vi "Sigma_SetSpeed.vi"(0 "VISA resource name":refnum<visa-resource-name>, 1 "Travel per Pulse (0.004mm)":dbl=0.004, 2 "Min (1mm) 2":dbl=1.0, 3 "Max (2mm) 2":dbl=2.0, 4 "Rate (1mm) 2":dbl=1.0, 5 "error in (no error)":errorcluster, 6 "Axis (1)":string="1", 8 "Min (1mm)":dbl=1.0, 10 "Max (2mm)":dbl=2.0, 12 "Rate (1mm)":dbl=1.0) -> (14 "VISA resource name out":refnum<visa-resource-name>, 19 "error out":errorcluster)   [LabVIEW 2018]
panel:
  out "resulting string":string
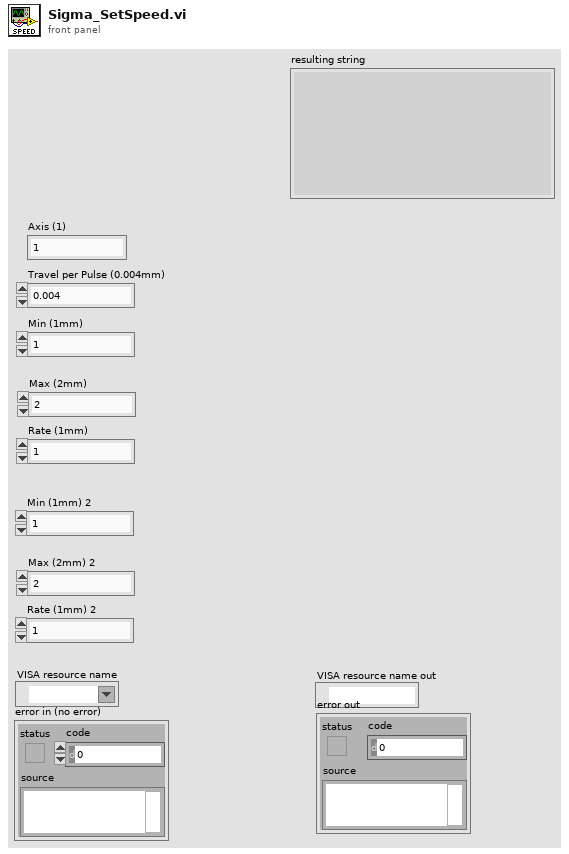
[diagram p1: front panel]
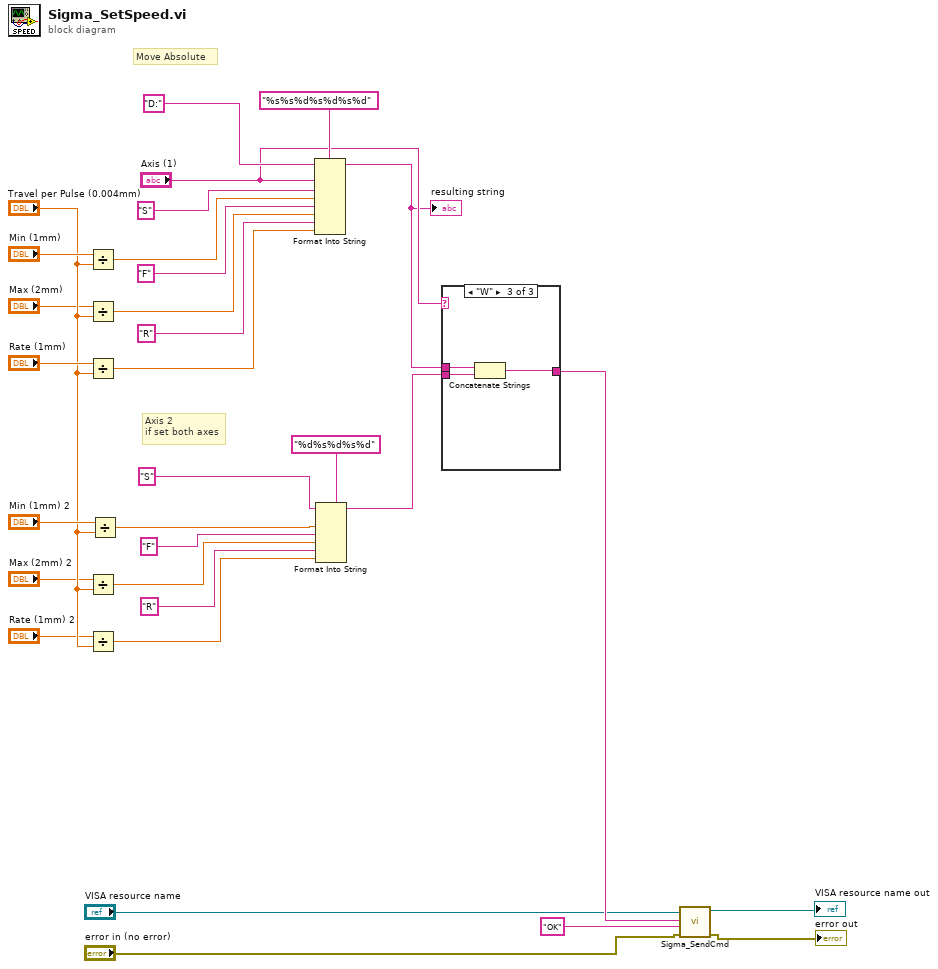
[diagram p0: block diagram]
diagram:
  # "Axis 2\nif set both axes"
  # "Move Absolute"
  n1 = Divide(x="Min (1mm)", y="Travel per Pulse (0.004mm)") -> (x/y=w18:dbl)
  n2 = Divide(x="Max (2mm)", y="Travel per Pulse (0.004mm)") -> (x/y=w13:dbl)
  n3 = Divide(x="Rate (1mm)", y="Travel per Pulse (0.004mm)") -> (x/y=w12:dbl)
  n4 = Divide(x="Max (2mm) 2", y="Travel per Pulse (0.004mm)") -> (x/y=w9:dbl)
  n5 = Divide(x="Rate (1mm) 2", y="Travel per Pulse (0.004mm)") -> (x/y=w7:dbl)
  n6 = Divide(x="Min (1mm) 2", y="Travel per Pulse (0.004mm)") -> (x/y=w11:dbl)
  n7 = Format Into String(format string="%s%s%d%s%d%s%d", initial string="D:" ("string"), "Axis (1)", "S" ("input 3"), w18, "F" ("input 3"), w13, "R" ("input 3"), w12) -> (resulting string=w20:string)  [unwired: 1 in, 1 out]
  "resulting string" <- w20
  n8 = Format Into String(format string="%d%s%d%s%d", initial string="S" ("input 3"), w11, "F" ("input 3"), w9, "R" ("input 3"), w7) -> (resulting string=w21:string)  [unwired: 1 in, 1 out]
  n9 = case shown="\"W\"" "Axis (1)" {
    tunnel: [w32 w33 w34] -> w6
    tunnel: w21 -> [_ w33 w35]
    tunnel: w20 -> [w32 _ w36]
    frame "1", Default {
    }
    frame "2" {
    }
    frame "W" {
      n10 = Concatenate Strings(w36, w35) -> (w34:string)
    }
  }
  n11 = call "Sigma_SendCmd.vi"("error in (no error)"="error in (no error)", "String to Receive"="OK", "String to Send"=w6, "VISA resource name"="VISA resource name") -> ("error out"=→"error out":errorcluster, "VISA resource name out"=→"VISA resource name out":refnum<visa-resource-name>)  [unwired: 4 in, 2 out]
